vi "Obtain Request Events.vi"(8 "error in":errorcluster, 10 "Create New? (F)":bool) -> (0 "error out":errorcluster, 2 "TS Environment Manager Request Events":T1)   [LabVIEW 2025, in "TS Environment Manager.lvlib"]
doc: "This VI Obtains/Creates the Requests events that will be used for other modules to communicate with the module that owns this VI. These Requests events will be accessed only via Public API methods for this module.\n\n<b>NOTE</b>: The contents of this VI are automatically generated and modified by the <b>Tools > DQMH Consortium > DQMH</b> utilities. Consider using those utilities instead of making your own modifications to this VI.\n_____\nBased on DQMH Dev Tools: Project Template 7.1.1.1528."
uses:
  TS Environment Manager.lvlib
  Request Events--cluster.ctl
  Stop Argument--cluster.ctl
  Show Panel Argument--cluster.ctl
  Hide Panel Argument--cluster.ctl
  Get Module Execution Status Argument--cluster.ctl
  Show Diagram Argument--cluster.ctl
  Get Installations Argument--cluster.ctl
  ITSDiscovery/ITSDiscovery.lvclass
  Get Installations (Reply Payload)--cluster.ctl
  Type Definitions/TSInstall--cluster.ctl
  Type Definitions/Architecture--enum.ctl
  Get Profiles File Argument--cluster.ctl
  Launch Sequence Editor Argument--cluster.ctl
  IProcess Executor/IProcess Executor.lvclass
  Launch Sequence Editor (Reply Payload)--cluster.ctl
  Activate Version Argument--cluster.ctl
  Activate Version (Reply Payload)--cluster.ctl
  Add Profile Argument--cluster.ctl
  Type Definitions/Profile--cluster.ctl
  Add Profile (Reply Payload)--cluster.ctl
  Get Profile(s) Argument--cluster.ctl
  Get Profile(s) (Reply Payload)--cluster.ctl
  Delete Profile Argument--cluster.ctl
  Delete Profile (Reply Payload)--cluster.ctl
  Set Profiles File Argument--cluster.ctl
  Set Profiles File (Reply Payload)--cluster.ctl
panel:
  # "NOTE: The contents of this VI are automatically generated and modified by the Tools > DQMH Consortium > DQMH utilities. Consider using those utilities instead of making your own modifications to this VI."
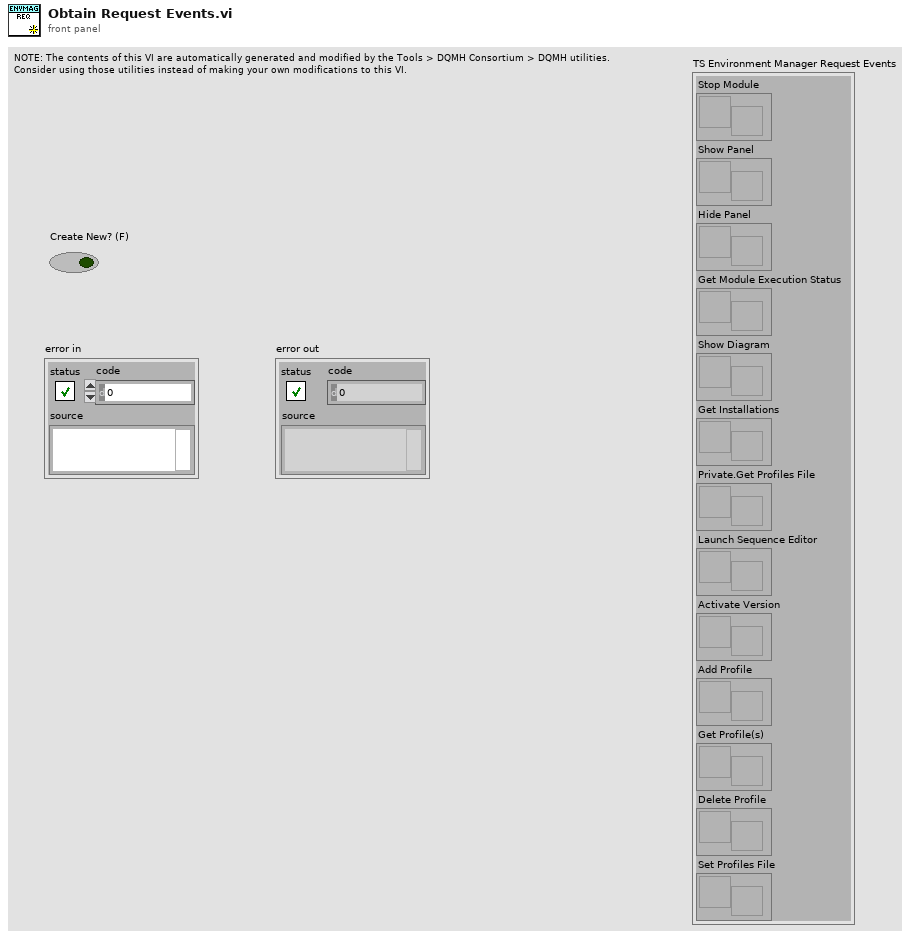
[diagram p1: front panel]
types:
  T1 = typedef "TS Environment Manager.lvlib/Request Events--cluster.ctl" = cluster{"Stop Module":refnum<user-event>, "Show Panel":refnum<user-event>, "Hide Panel":refnum<user-event>, "Get Module Execution Status":refnum<user-event>, "Show Diagram":refnum<user-event>, "Get Installations":refnum<user-event>, "Private.Get Profiles File":refnum<user-event>, "Launch Sequence Editor":refnum<user-event>, "Activate Version":refnum<user-event>, "Add Profile":refnum<user-event>, "Get Profile(s)":refnum<user-event>, "Delete Profile":refnum<user-event>, "Set Profiles File":refnum<user-event>}
  T2 = typedef "TS Environment Manager.lvlib/Set Profiles File Argument--cluster.ctl" = cluster{"File Path":path, "Wait Notifier":refnum<notifier>, "wait for reply":bool}
  T3 = typedef "TS Environment Manager.lvlib/Delete Profile Argument--cluster.ctl" = cluster{"Name":string, "Wait Notifier":refnum<notifier>, "wait for reply":bool}
  T4 = typedef "TS Environment Manager.lvlib/Get Profile(s) Argument--cluster.ctl" = cluster{"Name":string, "Wait Notifier":refnum<notifier>, "wait for reply":bool}
  T5 = typedef "TS Environment Manager.lvlib/Add Profile Argument--cluster.ctl" = cluster{"Profile":T6, "Wait Notifier":refnum<notifier>, "wait for reply":bool}
  T6 = typedef "Profile--cluster.ctl" = cluster{"Name":string, "Version":string, "Architecture":T7, "Environment":path}
  T7 = typedef "Architecture--enum.ctl" = enum16{"32bit", "64bit"}
  T8 = typedef "TS Environment Manager.lvlib/Activate Version Argument--cluster.ctl" = cluster{"Version":string, "IProcess Executor.lvclass":refnum<class "IProcess Executor.lvclass">, "ITSDiscovery.lvclass":refnum<class "ITSDiscovery.lvclass">, "Wait Notifier":refnum<notifier>, "wait for reply":bool}
  T9 = typedef "TS Environment Manager.lvlib/Launch Sequence Editor Argument--cluster.ctl" = cluster{"ITSDiscovery.lvclass":refnum<class "ITSDiscovery.lvclass">, "IProcess Executor.lvclass":refnum<class "IProcess Executor.lvclass">, "Version":string, "Architecture":T7, "Environment":path, "Wait Notifier":refnum<notifier>, "wait for reply":bool}
  T10 = typedef "TS Environment Manager.lvlib/Get Profiles File Argument--cluster.ctl" = cluster{"Boolean":bool}
  T11 = typedef "TS Environment Manager.lvlib/Get Installations Argument--cluster.ctl" = cluster{"ITSDiscovery.lvclass":refnum<class "ITSDiscovery.lvclass">, "Wait Notifier":refnum<notifier>, "wait for reply":bool}
  T12 = typedef "TS Environment Manager.lvlib/Hide Panel Argument--cluster.ctl" = cluster{"Hide Panel?":bool}
  T13 = typedef "TS Environment Manager.lvlib/Show Panel Argument--cluster.ctl" = cluster{"Show Panel?":bool}
  T14 = typedef "TS Environment Manager.lvlib/Show Diagram Argument--cluster.ctl" = cluster{"Debug?":bool}
  T15 = typedef "TS Environment Manager.lvlib/Get Module Execution Status Argument--cluster.ctl" = cluster{"Running?":bool}
  T16 = typedef "TS Environment Manager.lvlib/Stop Argument--cluster.ctl" = cluster{"Origin":string, "Exit via Stop Module Req?":bool, "Wait for Module to stop?":bool}
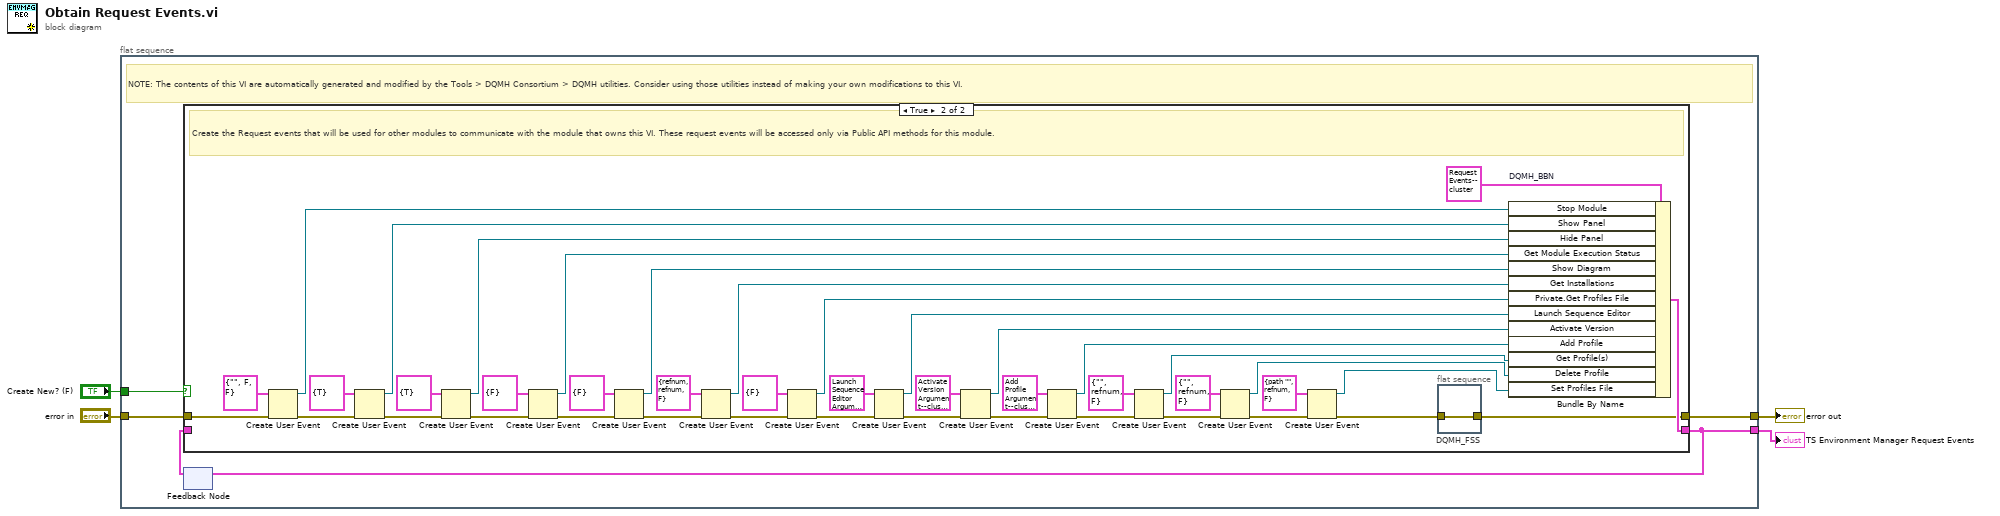
[diagram p0: block diagram]
diagram:
  n1 = flat-sequence {
    tunnel: [w9] -> w4
    tunnel: "error in" -> [w8]
    tunnel: [w6] -> w2
    tunnel: "Create New? (F)" -> [w5]
    frame #0 {
      # "NOTE: The contents of this VI are automatically generated and modified by the Tools > DQMH Consortium > DQMH utilities. Consider using those utilities instead of making your own modifications to this VI."
      n2 = feedback #1() -> (w7:T1)  [unwired: 1 in]
      n3 = case shown="True" w5 {
        tunnel: [w10 w44] -> w9
        tunnel: w8 -> [w10 w54]
        tunnel: [w11 w51] -> w6
        tunnel: w7 -> [w11 _]
        frame False {
          # "Obtain the Request events that were created in a previous call to this VI."
        }
        frame True {
          # "Create the Request events that will be used for other modules to communicate with the module that owns this VI. These request events will be accessed only via Public API methods for this module."
          n4 = Create User Event(user event datatype=T16 {"Origin"="", "Exit via Stop Module Req?"=FALSE, "Wait for Module to stop?"=FALSE} ("Stop Argument"), error in=w54) -> (user event=w52:refnum<user-event>, error out=w49:errorcluster)
          n5 = Create User Event(user event datatype=T13 {"Show Panel?"=TRUE} ("Show Panel Argument"), error in=w49) -> (user event=w48:refnum<user-event>, error out=w47:errorcluster)
          n6 = Create User Event(user event datatype=T12 {"Hide Panel?"=TRUE} ("Hide Panel Argument"), error in=w47) -> (user event=w46:refnum<user-event>, error out=w45:errorcluster)
          n7 = Create User Event(user event datatype=T15 {"Running?"=FALSE} ("Get Module Execution Status Argument"), error in=w45) -> (user event=w42:refnum<user-event>, error out=w43:errorcluster)
          n8 = Create User Event(user event datatype=T14 {"Debug?"=FALSE} ("Show Diagram Argument"), error in=w43) -> (user event=w39:refnum<user-event>, error out=w40:errorcluster)
          n9 = Create User Event(user event datatype=T11 {"ITSDiscovery.lvclass"=refnum, "Wait Notifier"=refnum, "wait for reply"=FALSE} ("Get Installations Argument"), error in=w40) -> (user event=w34:refnum<user-event>, error out=w35:errorcluster)
          n10 = Create User Event(user event datatype=T10 {"Boolean"=FALSE} ("Get Profile Argument"), error in=w35) -> (user event=w31:refnum<user-event>, error out=w32:errorcluster)
          n11 = Create User Event(user event datatype=T9 {"ITSDiscovery.lvclass"=refnum, "IProcess Executor.lvclass"=refnum, "Version"="", "Architecture"=enum."32bit", "Environment"=path "", "Wait Notifier"=refnum, "wait for reply"=FALSE} ("Launch Sequence Editor Argument"), error in=w32) -> (user event=w28:refnum<user-event>, error out=w29:errorcluster)
          n12 = Create User Event(user event datatype=T8 {"Version"="", "IProcess Executor.lvclass"=refnum, "ITSDiscovery.lvclass"=refnum, "Wait Notifier"=refnum, "wait for reply"=FALSE} ("Activate Version Argument"), error in=w29) -> (user event=w25:refnum<user-event>, error out=w26:errorcluster)
          n13 = Create User Event(user event datatype=T5 {"Profile"={"Name"="", "Version"="", "Architecture"=enum."32bit", "Environment"=path ""}, "Wait Notifier"=refnum, "wait for reply"=FALSE} ("Add Profile Argument"), error in=w26) -> (user event=w22:refnum<user-event>, error out=w23:errorcluster)
          n14 = Create User Event(user event datatype=T4 {"Name"="", "Wait Notifier"=refnum, "wait for reply"=FALSE} ("Get Profile(s) Argument"), error in=w23) -> (user event=w19:refnum<user-event>, error out=w20:errorcluster)
          n15 = Create User Event(user event datatype=T3 {"Name"="", "Wait Notifier"=refnum, "wait for reply"=FALSE} ("Delete Profile Argument"), error in=w20) -> (user event=w16:refnum<user-event>, error out=w17:errorcluster)
          n16 = Create User Event(user event datatype=T2 {"File Path"=path "", "Wait Notifier"=refnum, "wait for reply"=FALSE} ("Set Profiles File Argument"), error in=w17) -> (user event=w13:refnum<user-event>, error out=w14:errorcluster)
          n17 = flat-sequence "DQMH_FSS" {
            tunnel: w14 -> [w55]
            tunnel: [w55] -> w44
            frame #0 {
            }
          }
          n18 = Bundle By Name "DQMH_BBN"(cluster=T1 {"Stop Module"=refnum, "Show Panel"=refnum, "Hide Panel"=refnum, "Get Module Execution Status"=refnum, "Show Diagram"=refnum, "Get Installations"=refnum, "Private.Get Profiles File"=refnum, "Launch Sequence Editor"=refnum, "Activate Version"=refnum, "Add Profile"=refnum, "Get Profile(s)"=refnum, "Delete Profile"=refnum, "Set Profiles File"=refnum} ("output cluster"), "Stop Module"=w52, "Show Panel"=w48, "Hide Panel"=w46, "Get Module Execution Status"=w42, "Show Diagram"=w39, "Get Installations"=w34, "Private.Get Profiles File"=w31, "Launch Sequence Editor"=w28, "Activate Version"=w25, "Add Profile"=w22, "Get Profile(s)"=w19, "Delete Profile"=w16, "Set Profiles File"=w13) -> (w51:T1)
        }
      }
      n19 = feedback-in #1(w6) -> ()
    }
  }
  "TS Environment Manager Request Events" <- w2
  "error out" <- w4
